vi "New (Element).vi"(8 "error in (no error)":errorcluster, 10 "match behavior (keep)":T1, 11 "data item name":string) -> (0 "error out":errorcluster, 3 "data item out":refnum<class "Data Item.lvclass">)   [LabVIEW 2018, in "Logging.lvlib" / "Data Item.lvclass"]
uses:
  Data Item.lvclass
  extension/filter_interface/Match Behavior.ctl
  extension/filter_interface/Aggregation Method.ctl
  Logging.lvlib
panel:
  # "Connector Pane"
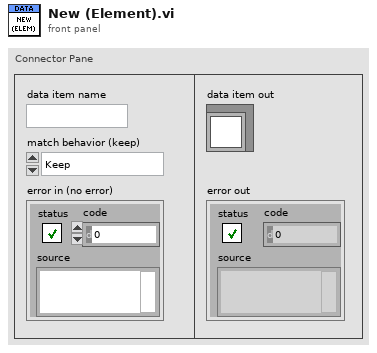
[diagram p1: front panel]
types:
  T1 = typedef "Logging.lvlib/Match Behavior.ctl" = enum16{"Keep", "Discard"}
  T2 = typedef "Logging.lvlib/Aggregation Method.ctl" = enum16{"Any", "Only", "All", "None"}
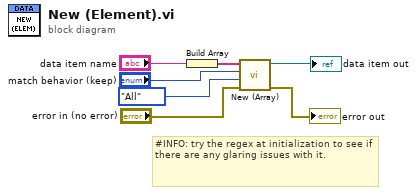
[diagram p0: block diagram]
diagram:
  # "#INFO: try the regex at initialization to see if there are any glaring issues with it."
  n1 = Build Array("data item name") -> (w6:string[])
  n2 = call "New (Array).vi"("error in (no error)"="error in (no error)", "aggregation method (all)"=Aggregation_Method."All" ("Method"), "match behavior (keep)"="match behavior (keep)", "data item names"=w6) -> ("error out"=→"error out":errorcluster, "data item out"=→"data item out":refnum<class "Data Item.lvclass">)  [unwired: 6 in]
